vi "submanueel.vi"(0 "links draaien":bool, 2 "achterwaarts":bool, 5 "rechts draaien":bool, 7 "snelheid":dbl, 9 "links draaien achteruit":bool, 12 "rechts draaien achteruit":bool, 13 "stoppen":bool, 14 "voorwaarts":bool) -> ()   [LabVIEW 2019]
uses:
  <vilib>/myRIO/Common/Instrument Driver Framework/Utilities/typedefs/Analog Scaling Constants.ctl
  <vilib>/myRIO/Common/Instrument Driver Framework/Utilities/typedefs/Analog Scaling Constants List.ctl
  <vilib>/myRIO/Common/Instrument Driver Framework/myRIO v1.0/AO/typedefs/AO Channels Enum.ctl
  <vilib>/myRIO/Common/Instrument Driver Framework/myRIO v1.0/AO/typedefs/AO Channels List.ctl
  <vilib>/myRIO/Common/Instrument Driver Framework/Utilities/typedefs/Generic FPGA Reference.ctl
  <vilib>/myRIO/Common/Instrument Driver Framework/Utilities/typedefs/myRIO v1.0 Reference.ctl
  <vilib>/myRIO/Common/Instrument Driver Framework/Utilities/typedefs/Hardware Version Enum.ctl
  <vilib>/myRIO/Common/Instrument Driver Framework/Utilities/typedefs/myRIO Generic Hardware Reference.ctl
  <vilib>/myRIO/Instrument Drivers/Onboard IO/AO/typedefs/AO Reference.ctl
  <vilib>/myRIO/Instrument Drivers/Onboard IO/AO/AO.lvlib
  <vilib>/myRIO/Instrument Drivers/Onboard IO/AO/vis/Write.vi
  <vilib>/userDefined/High Color/nirio_resource_hc.ctl
  <vilib>/myRIO/Common/Instrument Driver Framework/myRIO v1.0/AO/vis/myRIO v1.1 Open AO.vi
  <vilib>/myRIO/Instrument Drivers/Onboard IO/AO/vis/myRIO AO Open.xnode
  <vilib>/myRIO/Common/Instrument Driver Framework/Utilities/vis/Is FPGA Ref Available.vi
  <vilib>/myRIO/Express VI/Onboard IO/AO/AO Express VI.xnode
  subglobalbooleanmanueel.vi
panel:
  out "Boolean manueel":bool
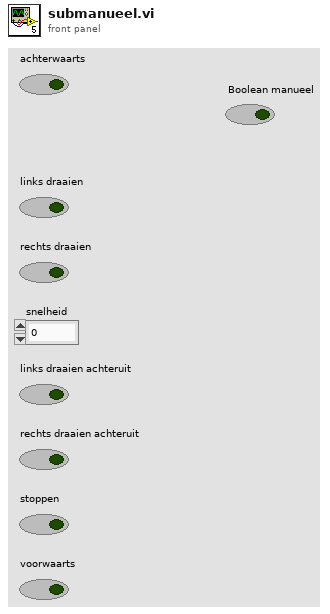
[diagram p1: front panel]
types:
  T1 = typedef "AO.lvlib/AO Reference.ctl" = cluster{"myRIO Reference":T2, "AO Channel List":T6, "AO Scaling Constant List":T8}
  T2 = typedef "myRIO Generic Hardware Reference.ctl" = cluster{"myRIO Model":T3, "myRIO Hardware Reference":T4}
  T3 = typedef "Hardware Version Enum.ctl" = enum16{"Unknown", "myRIO-1900", "myRIO-1950", "roboRIO", "NI ELVIS RIO CM", "ELVIS III"}
  T4 = typedef "myRIO v1.0 Reference.ctl" = cluster{"Generic FPGA Reference":T5, "Allow multiple opens":bool}
  T5 = typedef "Generic FPGA Reference.ctl" = refnum<k20>
  T6 = typedef "AO Channels List.ctl" = T7[]
  T7 = typedef "AO Channels Enum.ctl" = enum16{"Not Connected", "AudioOut/Left", "AudioOut/Right", "C/AO0", "C/AO1", "A/AO0", "A/AO1", "B/AO0", "B/AO1"}
  T8 = typedef "Analog Scaling Constants List.ctl" = T9[]
  T9 = typedef "Analog Scaling Constants.ctl" = cluster{"LSB Weight (Volts)":dbl, "Offset (Volts)":dbl, "Signed?":bool}
  T10 = typedef "nirio_resource_hc.ctl" = tag
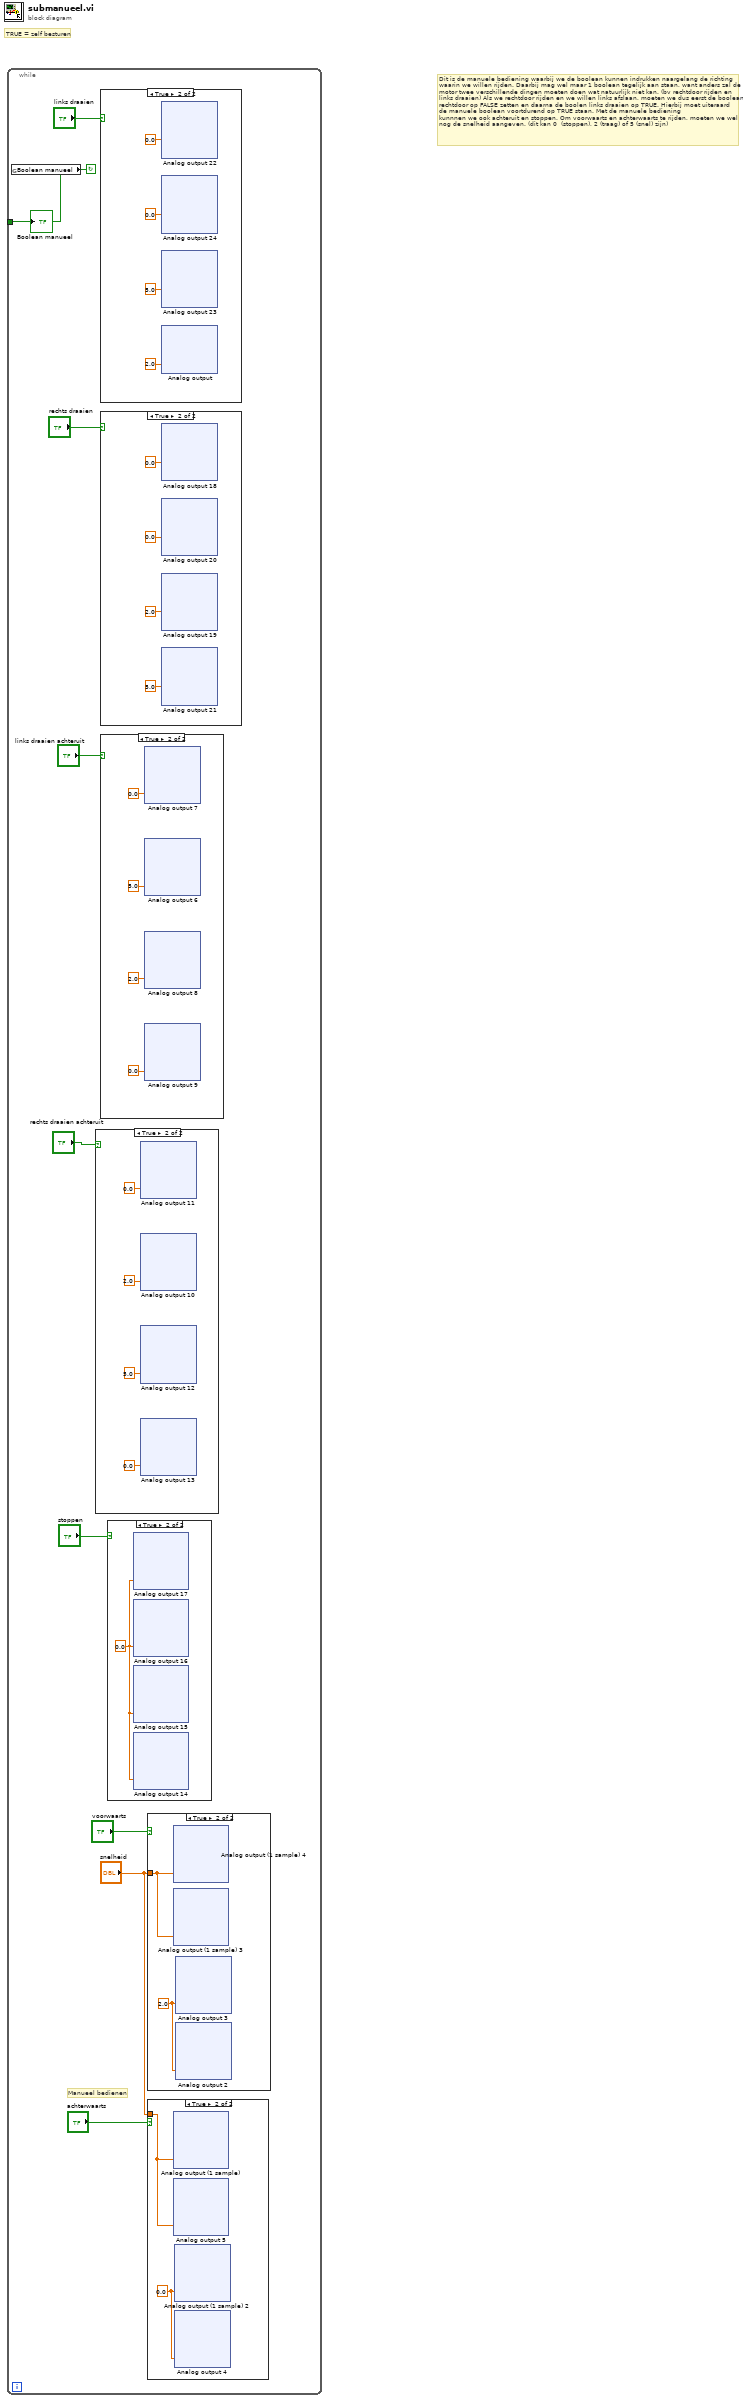
[diagram p0: block diagram]
diagram:
  # "TRUE = zelf besturen"
  # "Dit is de manuele bediening waarbij we de boolean kunnen indrukken naargelang de richting\nwaarin we willen rijden. Daarbij mag wel maar 1 boolean tegelijk aan staan, want anders zal de \nmotor twee verschillende dingen moeten doen wat natuurlijk niet kan. (bv rechtdoor rijden en\nlinks draaien) Als we rechtdoor rijden en we willen links afslaan, moeten we dus eerst de boolean\nrechtdoor op FALSE zetten en daarna de boolen links draaien op TRUE. Hierbij moet uiteraard\nde manuele boolean voortdurend op TRUE staan. Met de manuele bediening\nkunnnen we ook achteruit en stoppen. Om voorwaarts en achterwaarts te rijden, moeten we wel\nnog de snelheid aangeven. (dit kan 0  (stoppen), 2 (traag) of 5 (snel) zijn)"
  n1 = while {
    tunnel: [w1] -> _
    stop <- w1 continue-if-true
    # "Manueel bedienen"
    n2 = global read "subglobalbooleanmanueel.vi" "Boolean manueel"() -> (w1:bool)
    "Boolean manueel" <- w1
    n3 = case shown="True" "rechts draaien achteruit" {
      frame False {
      }
      frame True {
        n4 = xnode "Analog output 11"("B/AO0 (Pin 2)"=0.0) -> ()  [unwired: 1 in, 1 out]
        n5 = xnode "Analog output 10"("B/AO1 (Pin 4)"=2.0) -> ()  [unwired: 1 in, 1 out]
        n6 = xnode "Analog output 12"("A/AO1 (Pin 4)"=5.0) -> ()  [unwired: 1 in, 1 out]
        n7 = xnode "Analog output 13"("A/AO0 (Pin 2)"=0.0) -> ()  [unwired: 1 in, 1 out]
      }
    }
    n8 = case shown="True" "links draaien" {
      frame False {
      }
      frame True {
        n9 = xnode "Analog output 22"("B/AO1 (Pin 4)"=0.0) -> ()  [unwired: 1 in, 1 out]
        n10 = xnode "Analog output 24"("A/AO1 (Pin 4)"=0.0) -> ()  [unwired: 1 in, 1 out]
        n11 = xnode "Analog output 23"("B/AO0 (Pin 2)"=5.0) -> ()  [unwired: 1 in, 1 out]
        n12 = xnode "Analog output"("A/AO0 (Pin 2)"=2.0) -> ()  [unwired: 1 in, 1 out]
      }
    }
    n13 = case shown="True" "rechts draaien" {
      frame False {
      }
      frame True {
        n14 = xnode "Analog output 18"("B/AO1 (Pin 4)"=0.0) -> ()  [unwired: 1 in, 1 out]
        n15 = xnode "Analog output 20"("A/AO1 (Pin 4)"=0.0) -> ()  [unwired: 1 in, 1 out]
        n16 = xnode "Analog output 19"("B/AO0 (Pin 2)"=2.0) -> ()  [unwired: 1 in, 1 out]
        n17 = xnode "Analog output 21"("A/AO0 (Pin 2)"=5.0) -> ()  [unwired: 1 in, 1 out]
      }
    }
    n18 = case shown="True" "links draaien achteruit" {
      frame False {
      }
      frame True {
        n19 = xnode "Analog output 7"("B/AO0 (Pin 2)"=0.0) -> ()  [unwired: 1 in, 1 out]
        n20 = xnode "Analog output 6"("B/AO1 (Pin 4)"=5.0) -> ()  [unwired: 1 in, 1 out]
        n21 = xnode "Analog output 8"("A/AO1 (Pin 4)"=2.0) -> ()  [unwired: 1 in, 1 out]
        n22 = xnode "Analog output 9"("A/AO0 (Pin 2)"=0.0) -> ()  [unwired: 1 in, 1 out]
      }
    }
    n23 = case shown="True" "stoppen" {
      frame False {
      }
      frame True {
        w10 = 0.0
        n24 = xnode "Analog output 17"("A/AO0 (Pin 2)"=w10) -> ()  [unwired: 1 in, 1 out]
        n25 = xnode "Analog output 16"("A/AO1 (Pin 4)"=w10) -> ()  [unwired: 1 in, 1 out]
        n26 = xnode "Analog output 15"("B/AO0 (Pin 2)"=w10) -> ()  [unwired: 1 in, 1 out]
        n27 = xnode "Analog output 14"("B/AO1 (Pin 4)"=w10) -> ()  [unwired: 1 in, 1 out]
      }
    }
    n28 = case shown="True" "voorwaarts" {
      tunnel: "snelheid" -> [_ w917]
      frame False {
      }
      frame True {
        w918 = 2.0
        n29 = xnode "Analog output (1 sample) 4"("A/AO0 (Pin 2)"=w917) -> ()  [unwired: 1 in, 1 out]
        n30 = xnode "Analog output (1 sample) 3"("B/AO0 (Pin 2)"=w917) -> ()  [unwired: 1 in, 1 out]
        n31 = xnode "Analog output 3"("A/AO1 (Pin 4)"=w918) -> ()  [unwired: 1 in, 1 out]
        n32 = xnode "Analog output 2"("B/AO1 (Pin 4)"=w918) -> ()  [unwired: 1 in, 1 out]
      }
    }
    n33 = case shown="True" "achterwaarts" {
      tunnel: "snelheid" -> [_ w767]
      frame False {
      }
      frame True {
        w768 = 0.0
        n34 = xnode "Analog output (1 sample)"("A/AO1 (Pin 4)"=w767) -> ()  [unwired: 1 in, 1 out]
        n35 = xnode "Analog output 5"("B/AO1 (Pin 4)"=w767) -> ()  [unwired: 1 in, 1 out]
        n36 = xnode "Analog output (1 sample) 2"("A/AO0 (Pin 2)"=w768) -> ()  [unwired: 1 in, 1 out]
        n37 = xnode "Analog output 4"("B/AO0 (Pin 2)"=w768) -> ()  [unwired: 1 in, 1 out]
      }
    }
  }
